vi "motorIMU_csvReader_old.vi"() -> ()   [LabVIEW 2018]
uses:
  Control 12.ctl
  <vilib>/Instr/_visa.llb/VISA Configure Serial Port (Instr).vi
panel:
  in  "Tab Control":enum32{"VISA Config", "IMU", "Motor", "Errors"}(tab)
  in  "VISA":T1="COM4"
  in  "Timeout":u32=10000
  in  "termination char\n(0xA = '\\n' = LF)":u8 format="%.0x"
  in  "Enable Termination\nChar":bool=TRUE
  in  "data bits (8)":u16=8 min=5 max=8 step=1
  in  "parity (0:none)":enum16{"None", "Odd", "Even", "Mark", "Space"}(ring)
  in  "baud rate":u32=115200
  in  "y 2":bool
  in  "stop bits (10: 1 bit)":u16(ring)=10 items=["1.0"=10, "1.5"=15, "2.0"=20]
  out "Temperatura (ºC)":dbl(slide) scale=0.0..50.0 scale format="%#.2f"
  out "Acceleròmetre":cluster{dbl, dbl, dbl}(graph)={-1477.92, 1162.76, -1186.5} caption="Waveform Chart - Dark"
  out "Giroscòpi":cluster{dbl, dbl, dbl}(graph)={-1477.92, 1162.76, -1186.5} caption="Waveform Chart - Dark"
  out "Magnetometre":cluster{dbl, dbl, dbl}(graph)={-4031.37, -986.16, -4204.69} caption="Waveform Chart - Dark"
  in  "y":bool
  out "Bobina 3":bool
  out "Bobina 2":bool
  out "Bobina 1":bool
  out "Motor":cluster{"Data Out":dbl, "Data Out":dbl}(graph) caption="Waveform Chart - Dark"
  in  "y 3":bool
  out "Motor DataString":string
  out "Initial DataString":string
  out "error out":errorcluster
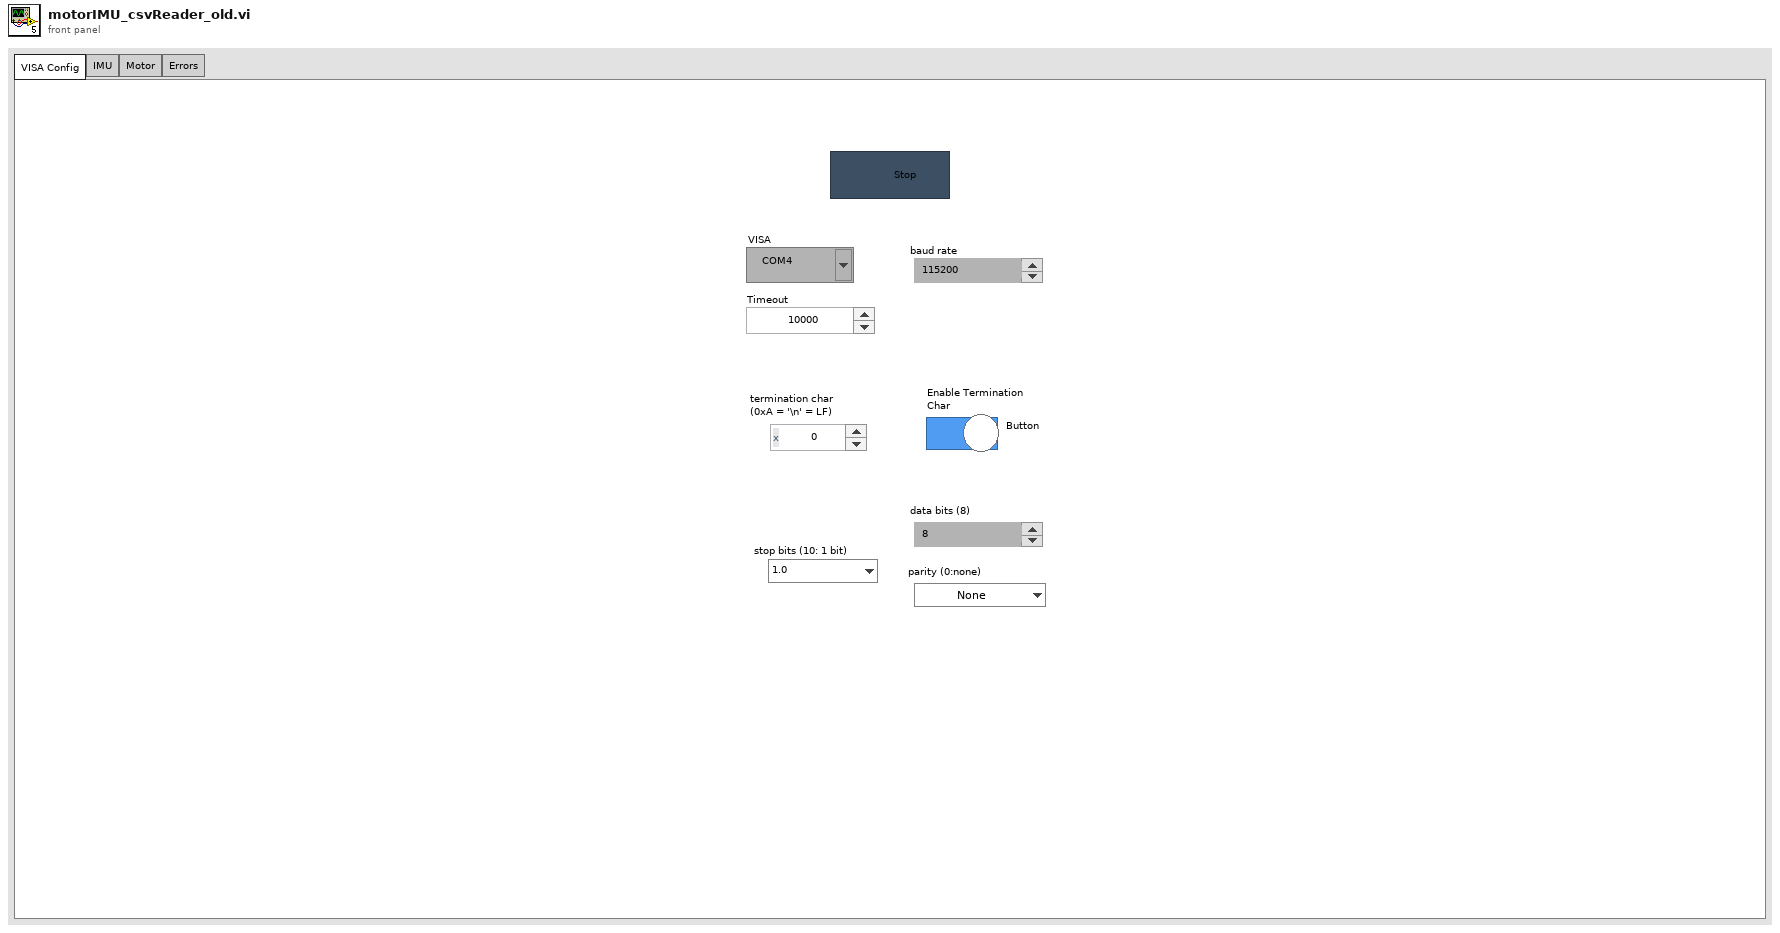
[diagram p1: front panel]
types:
  T1 = typedef "Control 12.ctl" = refnum<visa-resource-name>
  T2 = cluster{"Angle (graus)":dbl, "Fase (#bobina)":dbl}
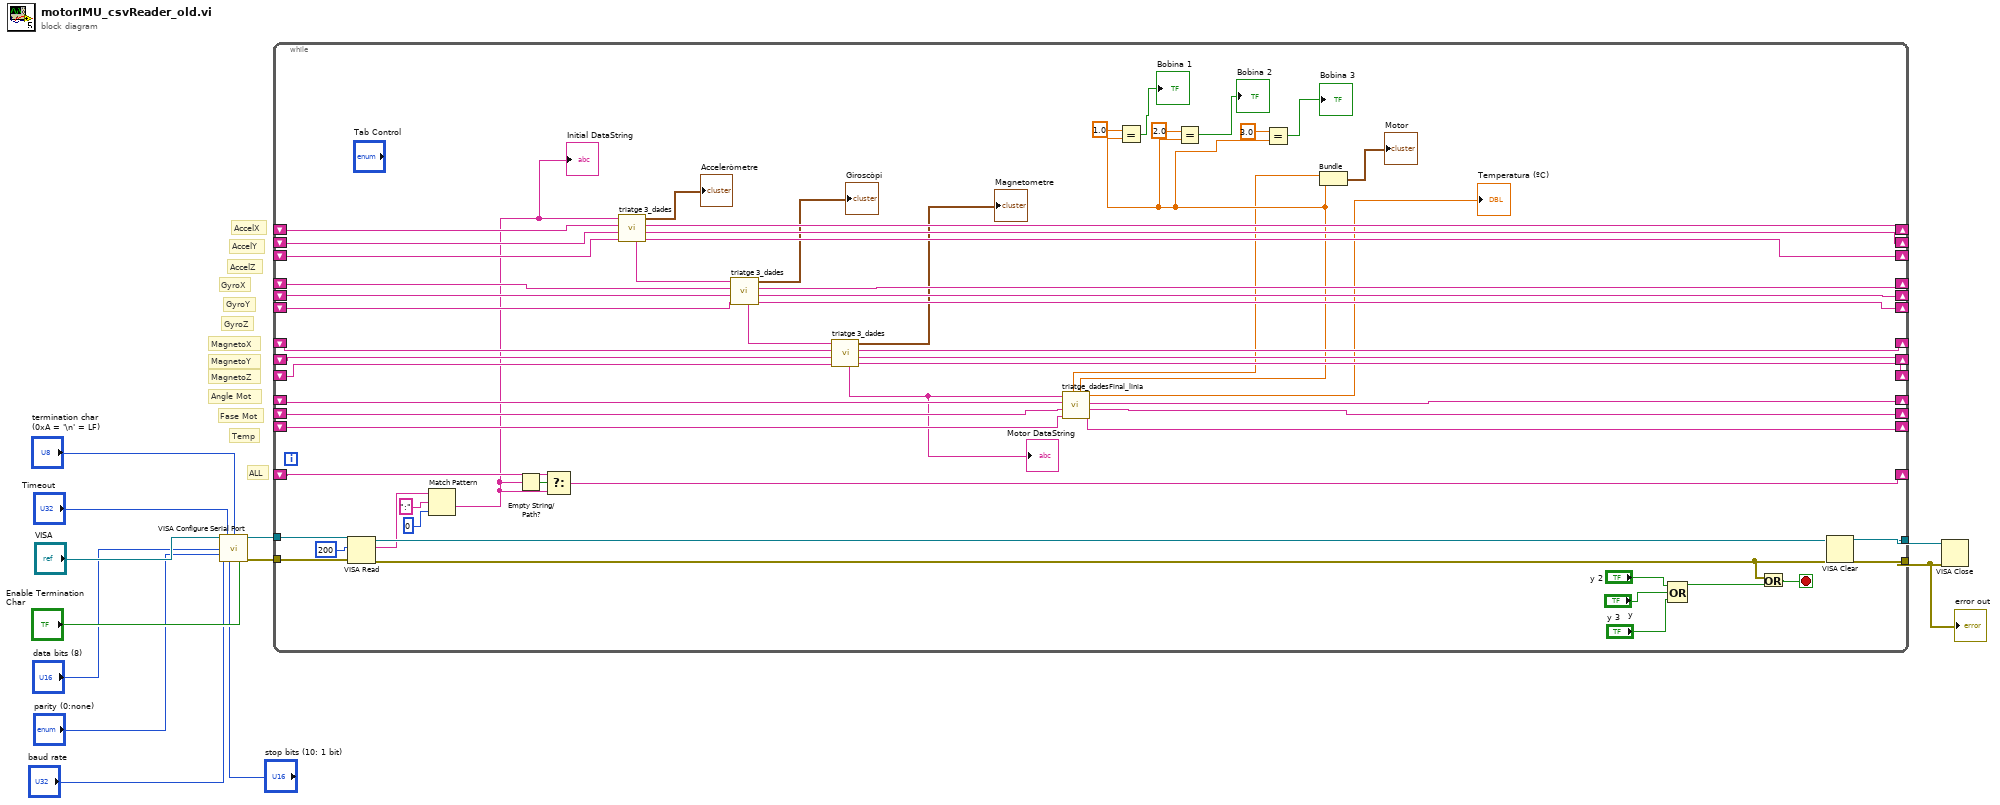
[diagram p0: block diagram]
diagram:
  # "Fase Mot"
  # "Angle Mot"
  # "ALL"
  # "Temp"
  # "MagnetoZ"
  # "MagnetoY"
  # "MagnetoX"
  # "GyroZ"
  # "AccelZ"
  # "GyroY"
  # "AccelY"
  # "GyroX"
  # "AccelX"
  n1 = call-poly "VISA Configure Serial Port"("VISA resource name"="VISA", "timeout (10sec)"="Timeout", "termination char\n(0xA = '\\n' = LF)"="termination char\n(0xA = '\\n' = LF)", "Enable Termination\nChar (T)"="Enable Termination\nChar", "baud rate (9600)"="baud rate", "data bits (8)"="data bits (8)", "parity (0:none)"="parity (0:none)", "stop bits (10: 1 bit)"="stop bits (10: 1 bit)") -> ("VISA resource name out"=w9:refnum<visa-resource-name>, "error out"=w7:errorcluster)  [unwired: 6 in]
  n2 = while {
    tunnel: w9 -> [w70]
    tunnel: [w69] -> w8
    tunnel: w7 -> [w68]
    tunnel: [w63] -> w6
    shift-right: [w48] -> _
    shift-left: _ -> [w49]
    shift-right: [w46] -> _
    shift-left: _ -> [w47]
    shift-right: [w36] -> _
    shift-left: _ -> [w37]
    shift-right: [w40] -> _
    shift-left: _ -> [w41]
    shift-right: [w38] -> _
    shift-left: _ -> [w39]
    shift-right: [w44] -> _
    shift-left: _ -> [w45]
    shift-right: [w28] -> _
    shift-left: _ -> [w29]
    shift-right: [w30] -> _
    shift-left: _ -> [w31]
    shift-right: [w32] -> _
    shift-left: _ -> [w33]
    shift-right: [w42] -> _
    shift-left: _ -> [w58]
    shift-right: [w27] -> _
    shift-left: _ -> [w26]
    shift-right: [w22] -> _
    shift-left: _ -> [w23]
    shift-right: [w25] -> _
    shift-left: _ -> [w24]
    stop <- w64 stop-if-true
    n3 = VISA Read(VISA resource name=w70, byte count=u32 200, error in (no error)=w68) -> (VISA resource name out=w69:refnum<visa-resource-name>, read buffer=w65:string, error out=w63:errorcluster)  [unwired: 1 out]
    n4 = Match Pattern(string=w65, regular expression=":", offset (0)=0 ("t")) -> (after substring=w16:string)  [unwired: 3 out]
    "Initial DataString" <- w16
    n5 = Empty String/Path?(string/path=w16) -> (empty?=w59:bool)
    n6 = Select(t=w58, s=w59, f=w16) -> (s? t:f=w42:string)
    n7 = call "triatge 3_dades.vi"("shift register left 3"=w45, "shift register left 2"=w47, "shift register left"=w49, "DataIN"=w16) -> ("shift register right 3"=w44:string, "shift register right 2"=w46:string, "shift register right"=w48:string, "Acceleròmetre"=→"Acceleròmetre":cluster{dbl, dbl, dbl}, "String Out"=w34:string)  [unwired: 3 in]
    n8 = call "triatge 3_dades.vi"("shift register left 3"=w37, "shift register left 2"=w39, "shift register left"=w41, "DataIN"=w34) -> ("shift register right 3"=w36:string, "shift register right 2"=w38:string, "shift register right"=w40:string, "Acceleròmetre"=→"Giroscòpi":cluster{dbl, dbl, dbl}, "String Out"=w15:string)  [unwired: 3 in]
    n9 = call "triatge 3_dades.vi"("shift register left 3"=w29, "shift register left 2"=w31, "shift register left"=w33, "DataIN"=w15) -> ("shift register right 3"=w28:string, "shift register right 2"=w30:string, "shift register right"=w32:string, "Acceleròmetre"=→"Magnetometre":cluster{dbl, dbl, dbl}, "String Out"=w17:string)  [unwired: 3 in]
    "Motor DataString" <- w17
    n10 = call "triatge_dadesFinal_linia.vi"("shift register left 3"=w23, "shift register left 2"=w24, "shift register left"=w26, "String in"=w17) -> ("shift register right 3"=w22:string, "shift register right 2"=w25:string, "shift register right"=w27:string, "Temp"=→"Temperatura (ºC)":dbl, "Fase (#bobina)"=w21:dbl, "Angle (graus)"=w20:dbl)  [unwired: 2 in]
    n11 = Equal?(x=1.0, y=w21) -> (x = y?=→"Bobina 1":bool)
    n12 = Equal?(x=2.0, y=w21) -> (x = y?=→"Bobina 2":bool)
    n13 = Equal?(x=3.0, y=w21) -> (x = y?=→"Bobina 3":bool)
    n14 = Bundle("Angle (graus)"=w20, "Fase (#bobina)"=w21) -> (→"Motor":T2)  [unwired: 1 in]
    n15 = Compound Arithmetic op=OR("y 2", "y", "y 3") -> (w60:bool)
    n16 = Or(x=w63, y=w60) -> (x .or. y?=w64:bool)
  }
  n17 = VISA Clear(VISA resource name=w8, error in (no error)=w6) -> (VISA resource name out=w10:refnum<visa-resource-name>, error out=w1:errorcluster)
  "error out" <- w1
  n18 = VISA Close(VISA resource name=w10, error in (no error)=w1) -> ()  [unwired: 1 out]
